vi "Delete Node From Dictionary.vi"(8 "error in (no error)":errorcluster, 10 "UID":string, 11 "Base Tree in":refnum<class "Base Tree.lvclass">) -> (0 "error out":errorcluster, 3 "Base Tree out":refnum<class "Base Tree.lvclass">)   [LabVIEW 2017, in "opcua.lvlib" / "Browser Core.lvlib" / "Base Tree.lvclass"]
doc: "Remove Node Class and Name pair from dictionary"
uses:
  Base Tree.lvclass
  Base Tree.lvclass/Base Tree.ctl
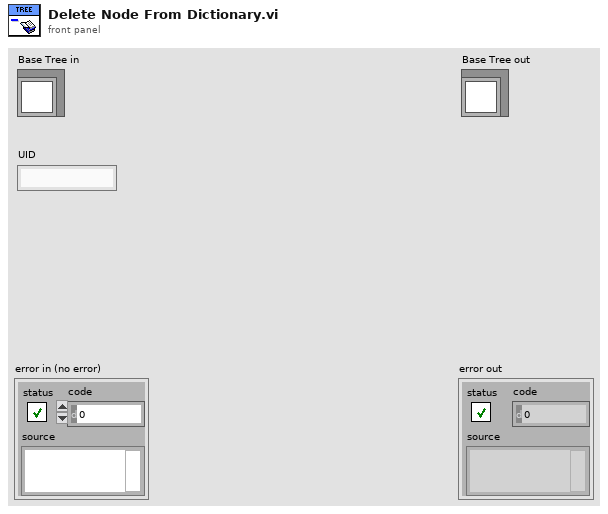
[diagram p1: front panel]
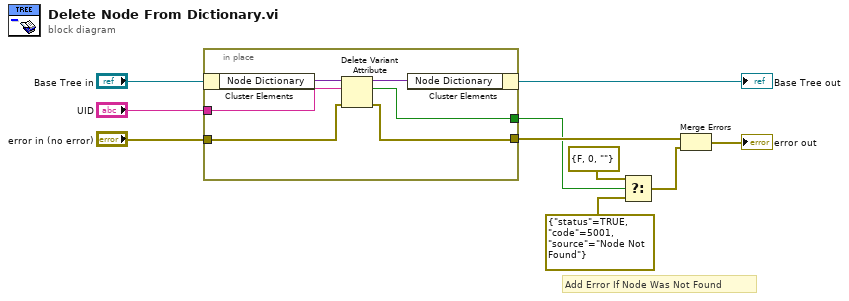
[diagram p0: block diagram]
diagram:
  # "Add Error If Node Was Not Found"
  n1 = in-place {
    in-place-border: "UID" -> [w15]
    in-place-border: "error in (no error)" -> [w13]
    in-place-border: [w12] -> w5
    in-place-border: [w11] -> w4
    n2 = in-place-cluster #1("Base Tree in") -> ("Node Dictionary"=w16:variant)
    n3 = Delete Variant Attribute(4:w13, 6:w15, 7:w16) -> (0:w12:errorcluster, 2:w11:bool, 3:w14:variant)
    n4 = in-place-cluster #1("Node Dictionary"=w14) -> (→"Base Tree out":refnum<class "Base Tree.lvclass">)
  }
  n5 = Select(t=errorcluster {"status"=FALSE, "code"=0, "source"=""}, s=w4, f=errorcluster {"status"=TRUE, "code"=5001, "source"="Node Not Found"} ("error IO")) -> (s? t:f=w1:errorcluster)
  n6 = Merge Errors(w5, w1) -> (→"error out":errorcluster)
